vi "Arrange Constant.vi"(8 "error in (no error)":errorcluster, 11 "GObject in":refnum<vi>) -> (0 "error out":errorcluster, 2 "object arranged?":bool, 3 "GObject out":refnum<vi>)   [LabVIEW 2019, in "Builtins.lvlib"]
doc: "Arranges the constant relative to the terminal position.\n\nCreated by: Ryan Pacini"
uses:
  <vilib>/Utility/miscctls.llb/LVPositionTypeDef.ctl
  Builtins.lvlib
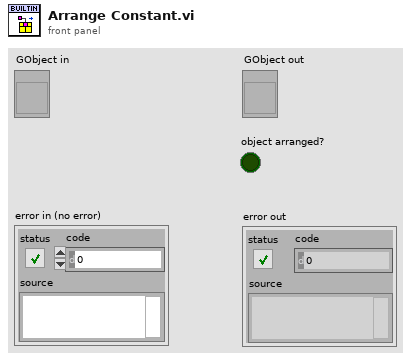
[diagram p1: front panel]
types:
  T1 = typedef "LVPositionTypeDef.ctl" = cluster{"Left":i32, "Top":i32}
  T2 = typedef "LVRectTypeDef.ctl" = cluster{"Left":i16, "Top":i16, "Right":i16, "Bottom":i16}
  T3 = cluster{"Left":i32, "Top":i32, "Right":i32, "Bottom":i32}
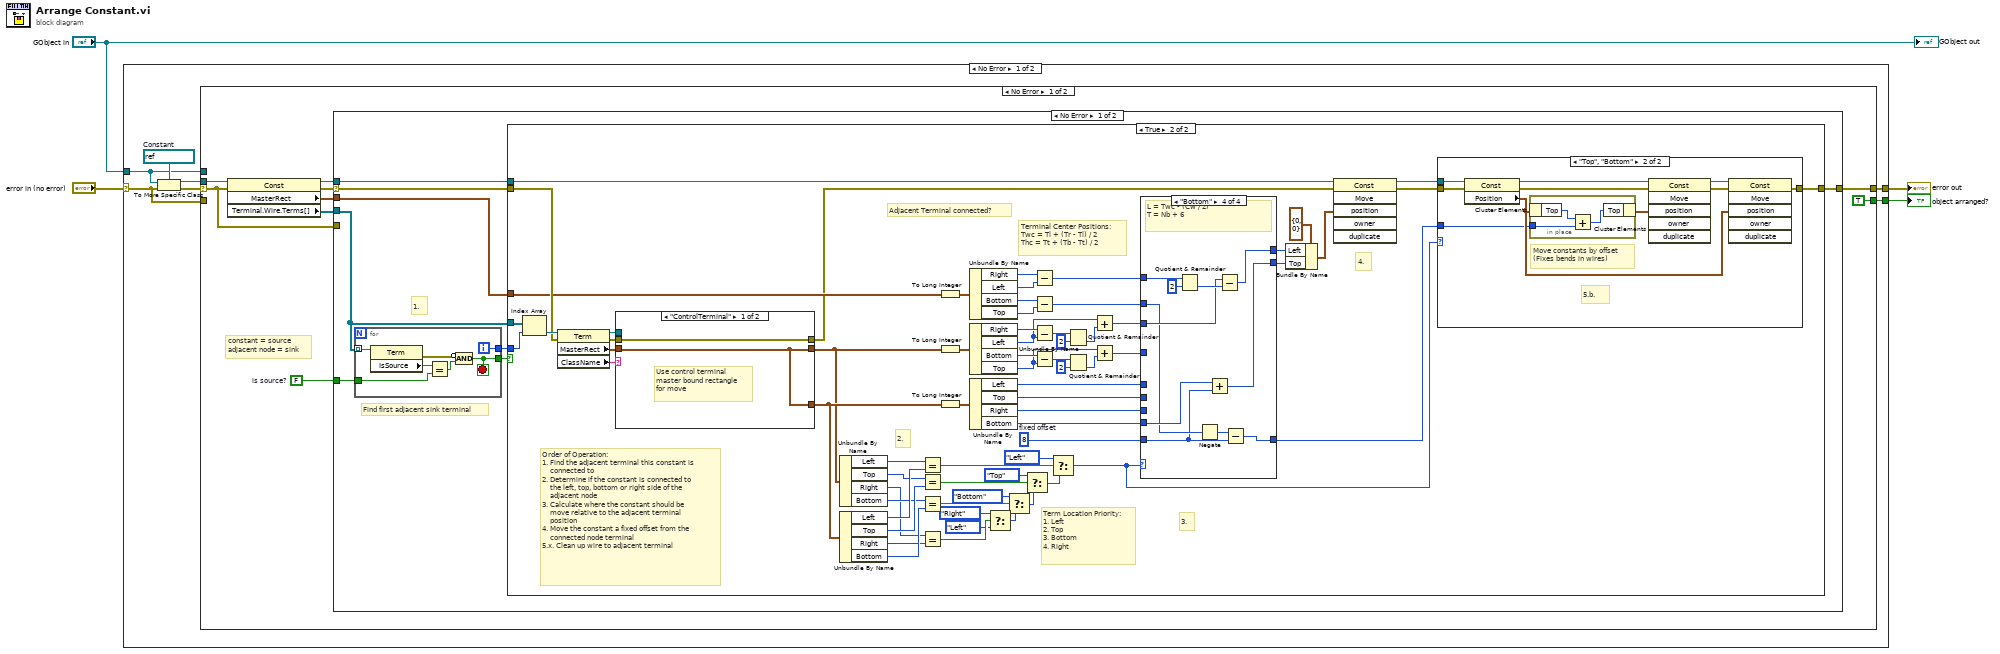
[diagram p0: block diagram]
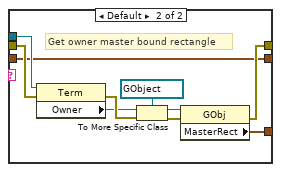
[diagram p3: hidden frame]
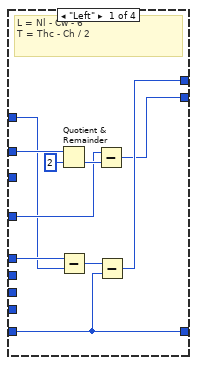
[diagram p4: hidden frame]
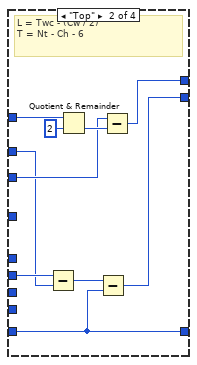
[diagram p5: hidden frame]
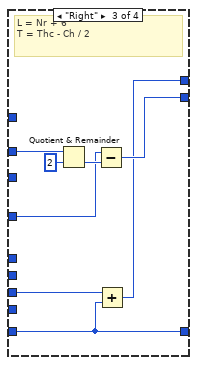
[diagram p6: hidden frame]
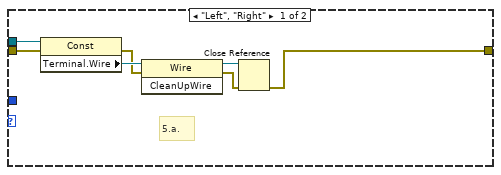
[diagram p7: hidden frame]
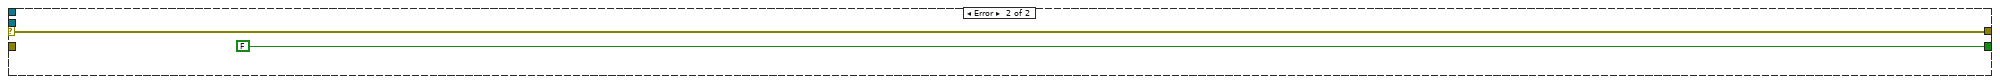
[diagram p9: hidden frame]
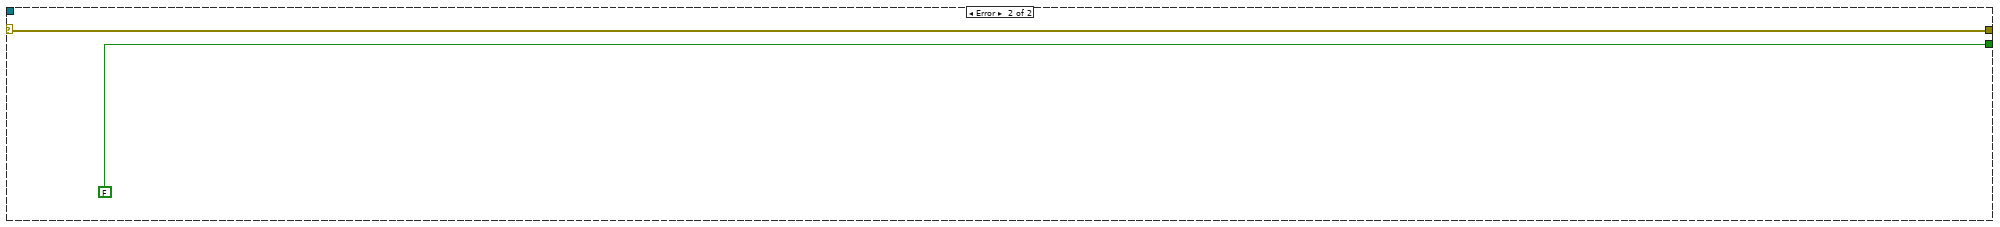
[diagram p10: hidden frame]
diagram:
  n1 = case shown="No Error" "error in (no error)" {
    selector: "error in (no error)" -> [w5 w180]
    tunnel: "GObject in" -> [w6 _]
    tunnel: [w11 w180] -> w2
    tunnel: [w10 FALSE] -> w1
    frame No Error {
      w9 = refnum<vi> refnum  # Constant
      n2 = To More Specific Class(target class=w9, reference=w6, error in=w5) -> (specific class reference=w7:refnum<vi>, error out=w8:errorcluster)
      n3 = case shown="No Error" w8 {
        selector: w8 -> [w12 _]
        tunnel: w7 -> [w19 _]
        tunnel: w6 -> [_ _]
        tunnel: w5 -> [_ w178]
        tunnel: [w15 w178] -> w11
        tunnel: [TRUE FALSE] -> w10
        frame No Error {
          w17 = FALSE  # is source?
          # "constant = source\nadjacent node = sink"
          n4 = property class="Const"(reference=w19, error in=w12) -> (reference out=w14:refnum<vi>, error out=w13:errorcluster, "MasterRect"=w16:T2, "Terminal.Wire.Terms[]"=w18:refnum<vi>[])
          n5 = case shown="No Error" w13 {
            selector: w13 -> [w21 _]
            tunnel: w18 -> [w28 _]
            tunnel: w17 -> [w27 _]
            tunnel: w16 -> [w24 _]
            tunnel: [w23 w176] -> w15
            tunnel: w14 -> [w22 _]
            tunnel: w12 -> [_ w176]
            frame No Error {
              # "1."
              # "Find first adjacent sink terminal"
              n6 = for {
                tunnel: w28 -> [w175] mode=indexing
                tunnel: [w174] -> w25
                tunnel: [w172] -> w26
                tunnel: w27 -> [w170]
                i -> [w174]
                stop <- w172 stop-if-true
                n7 = property class="Term"(reference=w175) -> (error out=w173:errorcluster, "IsSource"=w171:bool)  [unwired: 1 in, 1 out]
                n8 = Equal?(x=w171, y=w170) -> (x = y?=w169:bool)
                n9 = Compound Arithmetic op=AND(invert w173, w169) -> (w172:bool)
              }
              n10 = case shown="True" w26 {
                tunnel: w28 -> [_ w96]
                tunnel: w25 -> [_ w95]
                tunnel: w21 -> [w29 w94]
                tunnel: w24 -> [_ w73]
                tunnel: [w29 w40] -> w23
                tunnel: w22 -> [_ w42]
                frame False {
                }
                frame True {
                  w56 = 8  # fixed offset
                  # "Terminal Center Positions:\nTwc = Tl + (Tr - Tl) / 2\nThc = Tt + (Tb - Tt) / 2"
                  # "Order of Operation:\n1. Find the adjacent terminal this constant is \n    connected to\n2. Determine if the constant is connected to \n    the left, top, bottom or right side of the \n    adjacent node\n3. Calculate where the constant should be \n    move relative to the adjacent terminal\n    position\n4. Move the constant a fixed offset from the\n    connected node terminal \n5.x. Clean up wire to adjacent terminal"
                  # "4."
                  # "3."
                  # "2."
                  # "Term Location Priority:\n1. Left\n2. Top\n3. Bottom\n4. Right"
                  # "Adjacent Terminal connected?"
                  n11 = Index Array(array=w96, index=w95) -> (element=w97:refnum<vi>)
                  n12 = property class="Term"(reference=w97, error in=w94) -> (reference out=w33:refnum<vi>, error out=w34:errorcluster, "MasterRect"=w30:T2, "ClassName"=w32:string)
                  n13 = case shown="\"ControlTerminal\"" w32 {
                    tunnel: [w98 w106] -> w61
                    tunnel: [w99 w105] -> w41
                    tunnel: w34 -> [w99 w104]
                    tunnel: w33 -> [_ w102]
                    tunnel: [w98 w100] -> w31
                    tunnel: w30 -> [w98 w100]
                    frame "ControlTerminal" {
                      # "Use control terminal\nmaster bound rectangle\nfor move"
                    }
                    frame Default {
                      # "Get owner master bound rectangle"
                      n14 = property class="Term"(reference=w102, error in=w104) -> (error out=w103:errorcluster, "Owner"=w101:refnum<vi>)  [unwired: 1 out]
                      n15 = To More Specific Class(target class=refnum<vi> refnum ("Owner"), reference=w101, error in=w103) -> (specific class reference=w109:refnum<vi>, error out=w107:errorcluster)
                      n16 = property class="GObj"(reference=w109, error in=w107) -> (error out=w105:errorcluster, "MasterRect"=w106:T2)  [unwired: 1 out]
                    }
                  }
                  n17 = Unbundle By Name(w31) -> ("Left"=w93:i16, "Top"=w91:i16, "Right"=w79:i16, "Bottom"=w82:i16)
                  n18 = Unbundle By Name(w61) -> ("Left"=w92:i16, "Top"=w90:i16, "Right"=w78:i16, "Bottom"=w80:i16)
                  n19 = Equal?(x=w93, y=w92) -> (x = y?=w89:bool)
                  n20 = Equal?(x=w91, y=w90) -> (x = y?=w85:bool)
                  n21 = Equal?(x=w82, y=w80) -> (x = y?=w81:bool)
                  n22 = Equal?(x=w79, y=w78) -> (x = y?=w76:bool)
                  n23 = To Long Integer(number=w73) -> (32bit integer=w70:T3)
                  n24 = To Long Integer(number=w31) -> (32bit integer=w64:T3)
                  n25 = To Long Integer(number=w61) -> (32bit integer=w62:T3)
                  n26 = Unbundle By Name(w70) -> ("Right"=w71:i32, "Left"=w72:i32, "Bottom"=w69:i32, "Top"=w68:i32)
                  n27 = Unbundle By Name(w64) -> ("Right"=w63:i32, "Left"=w44:i32, "Bottom"=w65:i32, "Top"=w43:i32)
                  n28 = Unbundle By Name(w62) -> ("Left"=w60:i32, "Top"=w59:i32, "Right"=w58:i32, "Bottom"=w57:i32)
                  n29 = Select(t=enum8{"Left", "Top", "Right", "Bottom"}."Right" ("Location"), s=w76, f=enum8{"Left", "Top", "Right", "Bottom"}."Left" ("Location")) -> (s? t:f=w75:enum8{"Left", "Top", "Right", "Bottom"})
                  n30 = Select(t=enum8{"Left", "Top", "Right", "Bottom"}."Bottom" ("Location"), s=w81, f=w75) -> (s? t:f=w83:enum8{"Left", "Top", "Right", "Bottom"})
                  n31 = Select(t=enum8{"Left", "Top", "Right", "Bottom"}."Top" ("Location"), s=w85, f=w83) -> (s? t:f=w86:enum8{"Left", "Top", "Right", "Bottom"})
                  n32 = Subtract(x=w71, y=w72) -> (x-y=w67:i32)
                  n33 = Subtract(x=w69, y=w68) -> (x-y=w66:i32)
                  n34 = Subtract(x=w63, y=w44) -> (x-y=w49:i32)
                  n35 = Subtract(x=w65, y=w43) -> (x-y=w46:i32)
                  n36 = Select(t=enum8{"Left", "Top", "Right", "Bottom"}."Left" ("Location"), s=w89, f=w86) -> (s? t:f=w38:enum8{"Left", "Top", "Right", "Bottom"})
                  n37 = Quotient & Remainder(x=w49, y=2) -> (floor(x/y)=w50:i32)  [unwired: 1 out]
                  n38 = Quotient & Remainder(x=w46, y=2) -> (floor(x/y)=w37:i32)  [unwired: 1 out]
                  n39 = Add(x=w44, y=w50) -> (x+y=w48:i32)
                  n40 = Add(x=w43, y=w37) -> (x+y=w45:i32)
                  n41 = case shown="\"Bottom\"" w38 {
                    tunnel: [w112 w123 w131 w148] -> w55
                    tunnel: [w111 w124 w132 w143] -> w54
                    tunnel: w67 -> [w114 w128 _ w146]
                    tunnel: w66 -> [w117 w121 w135 w141]
                    tunnel: w48 -> [_ w122 _ w144]
                    tunnel: w45 -> [w116 _ w134 _]
                    tunnel: w60 -> [w115 _ _ _]
                    tunnel: w59 -> [_ w126 _ _]
                    tunnel: w58 -> [_ _ w133 _]
                    tunnel: w57 -> [_ _ _ w142]
                    tunnel: w56 -> [w110 w120 w130 w138]
                    tunnel: [w110 w120 w130 w140] -> w39
                    frame "Left" {
                      # "L = Nl - Cw - 6\nT = Thc - Ch / 2"
                      n42 = Quotient & Remainder(x=w117, y=2) -> (floor(x/y)=w118:i32)  [unwired: 1 out]
                      n43 = Subtract(x=w115, y=w114) -> (x-y=w113:i32)
                      n44 = Subtract(x=w116, y=w118) -> (x-y=w111:i32)
                      n45 = Subtract(x=w113, y=w110) -> (x-y=w112:i32)
                    }
                    frame "Top" {
                      # "L = Twc - (Cw / 2)\nT = Nt - Ch - 6"
                      n46 = Subtract(x=w126, y=w121) -> (x-y=w125:i32)
                      n47 = Quotient & Remainder(x=w128, y=2) -> (floor(x/y)=w127:i32)  [unwired: 1 out]
                      n48 = Subtract(x=w125, y=w120) -> (x-y=w124:i32)
                      n49 = Subtract(x=w122, y=w127) -> (x-y=w123:i32)
                    }
                    frame "Right" {
                      # "L = Nr + 6\nT = Thc - Ch / 2"
                      n50 = Quotient & Remainder(x=w135, y=2) -> (floor(x/y)=w136:i32)  [unwired: 1 out]
                      n51 = Subtract(x=w134, y=w136) -> (x-y=w132:i32)
                      n52 = Add(x=w133, y=w130) -> (x+y=w131:i32)
                    }
                    frame "Bottom" {
                      # "L = Twc - (Cw / 2)\nT = Nb + 6"
                      n53 = Quotient & Remainder(x=w146, y=2) -> (floor(x/y)=w145:i32)  [unwired: 1 out]
                      n54 = Negate(x=w141) -> (-x=w139:i32)
                      n55 = Add(x=w142, y=w138) -> (x+y=w143:i32)
                      n56 = Subtract(x=w144, y=w145) -> (x-y=w148:i32)
                      n57 = Subtract(x=w139, y=w138) -> (x-y=w140:i32)
                    }
                  }
                  n58 = Bundle By Name(cluster=T1 {"Left"=0, "Top"=0} ("Position"), "Left"=w55, "Top"=w54) -> (w52:T1)
                  n59 = invoke class="Const" method="Move"(reference=w42, error in=w41, "position"=w52) -> (reference out=w35:refnum<vi>, error out=w36:errorcluster)  [unwired: 3 in, 4 out]
                  n60 = case shown="\"Top\", \"Bottom\"" w38 {
                    tunnel: w35 -> [w152 w165]
                    tunnel: w36 -> [w149 w156]
                    tunnel: [w150 w161] -> w40
                    tunnel: w39 -> [_ w158]
                    frame "Left", "Right" {
                      # "5.a."
                      n61 = property class="Const"(reference=w152, error in=w149) -> (error out=w151:errorcluster, "Terminal.Wire"=w155:refnum<vi>)  [unwired: 1 out]
                      n62 = invoke class="Wire" method="CleanUpWire"(reference=w155, error in=w151) -> (reference out=w154:refnum<vi>, error out=w153:errorcluster)  [unwired: 1 in, 1 out]
                      n63 = Close Reference(reference=w154, error in (no error)=w153) -> (error out=w150:errorcluster)
                    }
                    frame "Top", "Bottom" {
                      # "5.b."
                      # "Move constants by offset\n(Fixes bends in wires)"
                      n64 = property class="Const"(reference=w165, error in=w156) -> (reference out=w164:refnum<vi>, error out=w163:errorcluster, "Position"=w159:T1)
                      n65 = in-place {
                        in-place-border: w158 -> [w166]
                        n66 = in-place-cluster #1(w159) -> ("Top"=w168:i32)
                        n67 = Add(x=w168, y=w166) -> (x+y=w167:i32)
                        n68 = in-place-cluster #1("Top"=w167) -> (w162:T1)
                      }
                      n69 = invoke class="Const" method="Move"(reference=w164, error in=w163, "position"=w162) -> (reference out=w160:refnum<vi>, error out=w157:errorcluster)  [unwired: 3 in, 4 out]
                      n70 = invoke class="Const" method="Move"(reference=w160, error in=w157, "position"=w159) -> (error out=w161:errorcluster)  [unwired: 3 in, 5 out]
                    }
                  }
                }
              }
            }
            frame Error {
              # "No wires connected"
            }
          }
        }
        frame Error {
        }
      }
    }
    frame Error {
    }
  }
  "error out" <- w2
  "object arranged?" <- w1
  "GObject out" <- "GObject in"
